vi "Set Angle.vi"(6 "Axis":T1, 8 "error in (no error)":errorcluster, 9 "Rate (°/min)":dbl, 10 "Angle (°)":dbl, 11 "Inst.Xeryon-Rotator in":refnum<class "Inst.Xeryon-Rotator.lvclass">) -> (0 "error out":errorcluster, 3 "Inst.Xeryon-Rotator out":refnum<class "Inst.Xeryon-Rotator.lvclass">)   [LabVIEW 2019, in "Inst.Xeryon-Rotator.lvclass"]
uses:
  Inst.Xeryon-Rotator.lvclass
  C:/Program Files (x86)/National Instruments/LabVIEW 2019/user.lib/LevyLab/Instrument Framework/Instrument/Instrument.lvclass
  Typedefs/Inst.Xeryon-Rotator.Commands--Enum.ctl
  <userlib>/LevyLab/Instrument Framework/Instrument/Instrument.lvclass
  <userlib>/LevyLab/Instrument Framework/Instrument Types/Cryostat/Typedefs/setAngle--cluster.ctl
  <userlib>/LevyLab/Instrument Framework/Instrument Types/Cryostat/Instrument.Cryostat.lvclass
  <userlib>/LevyLab/Instrument Framework/Instrument Types/Cryostat/Typedefs/Rotator Axis--Enum.ctl
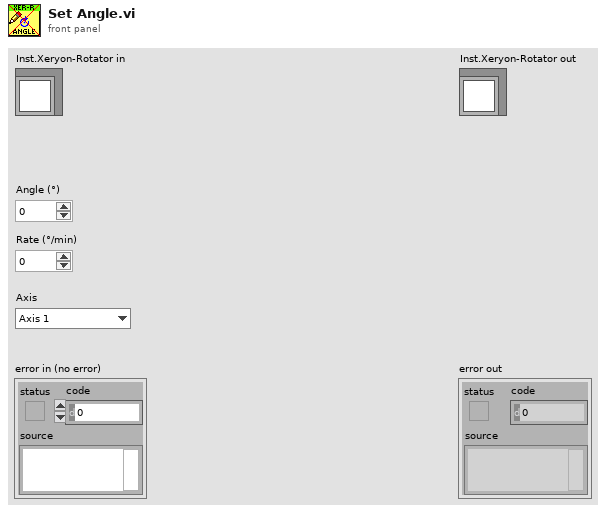
[diagram p1: front panel]
types:
  T1 = typedef "Instrument.Cryostat.lvclass/Rotator Axis--Enum.ctl" = enum16{"Axis 1", "Axis 2"}
  T2 = typedef "Instrument.Cryostat.lvclass/setAngle--cluster.ctl" = cluster{"angle":dbl, "rate":dbl, "channel":i32}
  T3 = typedef "Inst.Xeryon-Rotator.lvclass/Inst.Xeryon-Rotator.Commands--Enum.ctl" = enum16{"setAngle", "getAngle", "setState"}
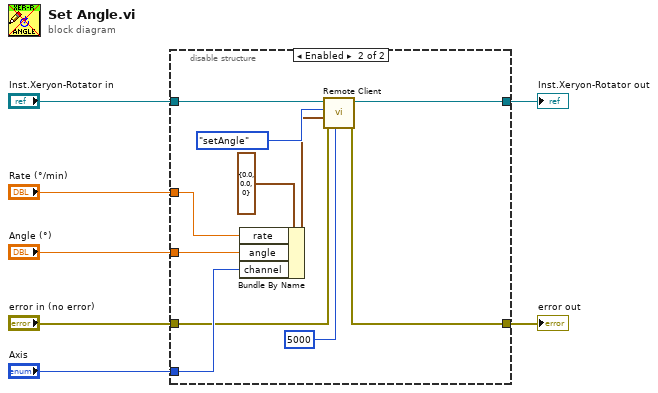
[diagram p0: block diagram]
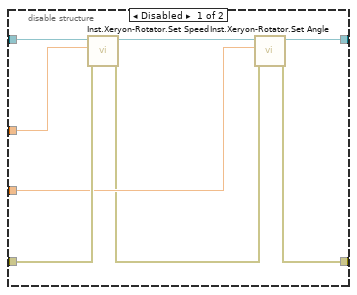
[diagram p2: hidden frame]
diagram:
  n1 = disable-structure shown="Enabled" {
    disable-tunnel: "Inst.Xeryon-Rotator in" -> [w15 w26]
    disable-tunnel: "Rate (°/min)" -> [w13 w22]
    disable-tunnel: "error in (no error)" -> [w12 w20]
    disable-tunnel: "Angle (°)" -> [w11 w23]
    disable-tunnel: [w10 w17] -> w3
    disable-tunnel: [w9 w18] -> w2
    disable-tunnel: "Axis" -> [_ w21]
    frame Disabled {
      n2 = call "Inst.Xeryon-Rotator.Set Speed.vi"("error in (no error)"=w12, "Rate (°/min)"=w13, "Inst.Xeryon-Rotator in"=w15) -> ("error out"=w8:errorcluster, "Inst.Xeryon-Rotator out"=w14:refnum<class "Inst.Xeryon-Rotator.lvclass">)  [unwired: 7 in]
      n3 = call "Inst.Xeryon-Rotator.Set Angle.vi"("error in (no error)"=w8, "Angle (°)"=w11, "Inst.Xeryon-Rotator in"=w14) -> ("error out"=w9:errorcluster, "Inst.Xeryon-Rotator out"=w10:refnum<class "Inst.Xeryon-Rotator.lvclass">)  [unwired: 7 in]
    }
    frame Enabled {
      n4 = Bundle By Name(cluster=T2 {"angle"=0.0, "rate"=0.0, "channel"=0} ("setAngle"), "rate"=w22, "angle"=w23, "channel"=w21) -> (w19:T2)
      n5 = call <userlib>:"Remote Client.vi"("timeout (ms) [500]"=5000, "error in (no error)"=w20, "Data in"=w19, "Command in"=Inst.Xeryon-Rotator.Commands--Enum."setAngle" ("Commands"), "Instrument in"=w26) -> ("error out"=w18:errorcluster, "Instrument out"=w17:refnum<class "Inst.Xeryon-Rotator.lvclass">)  [unwired: 3 in, 2 out]
    }
  }
  "error out" <- w2
  "Inst.Xeryon-Rotator out" <- w3
